vi "Variant to Dictionary.vi"(8 "error in (no error)":errorcluster, 11 "Array in":cluster{"Data (Dictionary)":T1[]}[](array[cluster])) -> (0 "error out":errorcluster, 3 "Array out":cluster{"Data (Dictionary)":T1[]}[](array[cluster]))   [LabVIEW 2019, in "LV-Data.lvclass"]
doc: "This VI is meant to reconcile several data formats:\n\ni. Array (1) of Cluster of Array of Dictionary [Key, Dictionary [Key, Data Array]] (e.g. all data in 1 TDMS file)\nii. Array (N) of Cluster of Array of Dictionary [Key, Dictionary [Key, Data Array]] (e.g. data in folder of TDMS files)\niii. Array (1) of Cluster of Array of Dictionary [Key, Data Array] (e.g. data in dat file)"
uses:
  LV-Data.lvclass
  Typedefs/Dictionary--cluster.ctl
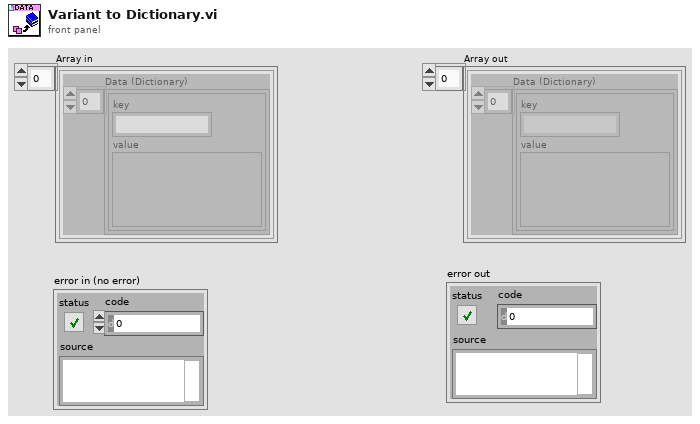
[diagram p1: front panel]
types:
  T1 = typedef "LV-Data.lvclass/Dictionary--cluster.ctl" = cluster{"key":string, "value":variant}
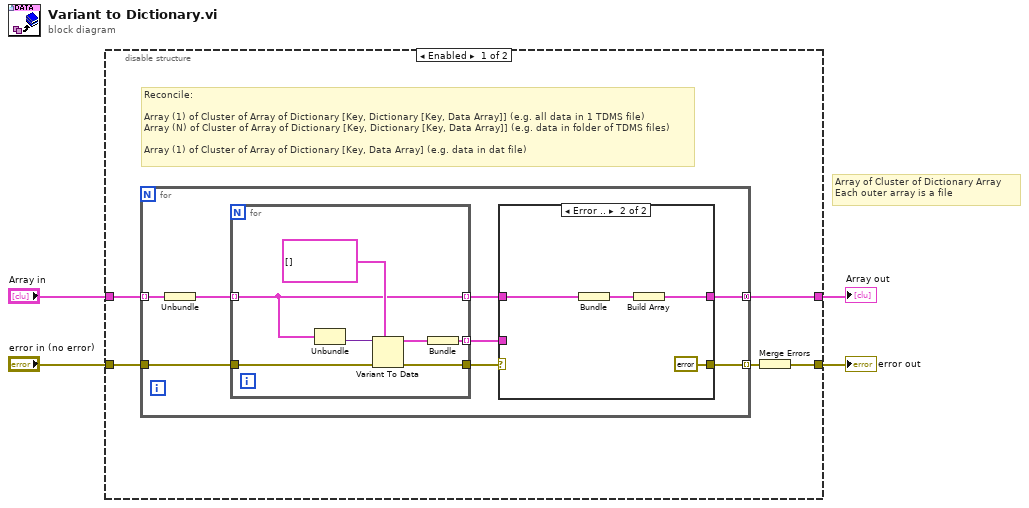
[diagram p0: block diagram]
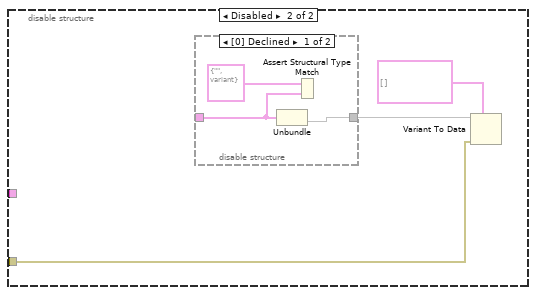
[diagram p3: hidden frame]
diagram:
  # "Array of Cluster of Dictionary Array\nEach outer array is a file"
  n1 = disable-structure shown="Enabled" {
    disable-tunnel: "Array in" -> [w9 _]
    disable-tunnel: [w7 _] -> w4
    disable-tunnel: [w6 _] -> w3
    disable-tunnel: "error in (no error)" -> [w5 w31]
    frame Enabled {
      # "Reconcile: \n\nArray (1) of Cluster of Array of Dictionary [Key, Dictionary [Key, Data Array]] (e.g. all data in 1 TDMS file)\nArray (N) of Cluster of Array of Dictionary [Key, Dictionary [Key, Data Array]] (e.g. data in folder of TDMS files)\n\nArray (1) of Cluster of Array of Dictionary [Key, Data Array] (e.g. data in dat file)"
      n2 = for {
        tunnel: w9 -> [w17] mode=indexing
        tunnel: [w13] -> w6 mode=concatenating
        tunnel: [w12] -> w8 mode=indexing
        tunnel: w5 -> [w10]
        n3 = Unbundle(w17) -> ("Data (Dictionary)"=w16:T1[])
        n4 = for {
          tunnel: [w30] -> w15
          tunnel: w16 -> [w25] mode=indexing
          tunnel: [w27] -> w14 mode=indexing
          tunnel: [w25] -> w11 mode=indexing
          tunnel: w10 -> [w24]
          n5 = Unbundle(w25) -> ("value"=w29:variant)  [unwired: 1 out]
          n6 = Variant To Data(error in=w24, type=T1[] [] ("Array"), Variant=w29) -> (data=w28:T1[], error out=w30:errorcluster)
          n7 = Bundle("Array"=w28) -> (w27:cluster{"Array":T1[]})  [unwired: 1 in]
        }
        n8 = case shown="Error .." w15 {
          selector: w15 -> [w18 _]
          tunnel: w14 -> [w19 _]
          tunnel: [w19 w21] -> w13
          tunnel: [w18 errorcluster {"status"=FALSE, "code"=0, "source"=""} ("error IO")] -> w12
          tunnel: w11 -> [_ w23]
          frame No Error {
          }
          frame Error {
            n9 = Bundle(w23) -> (w22:cluster{T1[]})  [unwired: 1 in]
            n10 = Build Array(w22) -> (w21:cluster{T1[]}[])
          }
        }
      }
      n11 = Merge Errors(w8) -> (w7:errorcluster)
    }
    frame Disabled {
      n12 = disable-structure shown="[0] Declined" {
        disable-tunnel: [w36 w38] -> w33
        disable-tunnel: [w35 w38] -> w34
        frame Disabled {
          n13 = Unbundle(w35) -> ("value"=w36)  [unwired: 1 out]
          n14 = Assert Structural Type Match(0:w35, 1:T1 {"key"="", "value"=variant} ("key-value")) -> ()
        }
        frame Enabled {
        }
      }
      n15 = Variant To Data(error in=w31, type=T1[] [] ("Array"), Variant=w33) -> ()  [unwired: 2 out]
    }
  }
  "error out" <- w4
  "Array out" <- w3
